vi "stop.vi"(8 "error in (no error)":errorcluster, 11 "SignalReaderCN091129DAQmx in":refnum<class "SignalReaderCN091129DAQmx.lvclass">) -> (0 "error out":errorcluster, 3 "SignalReaderCN091129DAQmx out":refnum<class "SignalReaderCN091129DAQmx.lvclass">)   [LabVIEW 2010, in "SignalReaderCN091129DAQmx.lvclass"]
uses:
  SignalReaderCN091129DAQmx.lvclass
  GenericSignalReader/GenericSignalReader/GenericSignalReader.lvclass
  SignalReaderCN091129DAQmx.lvclass/SignalReaderCN091129DAQmx.ctl
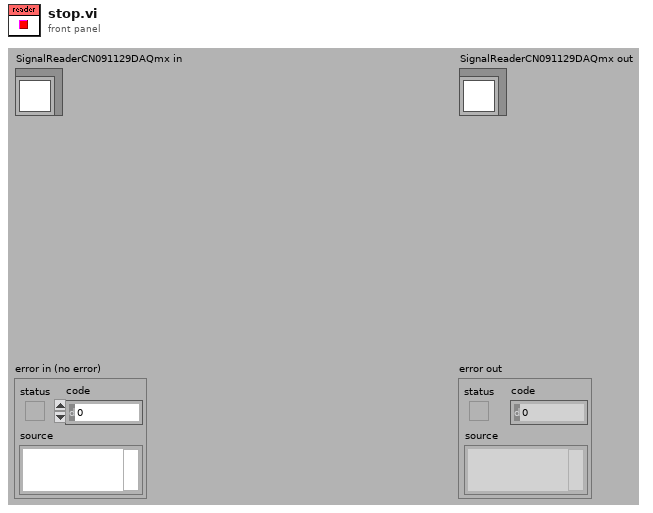
[diagram p1: front panel]
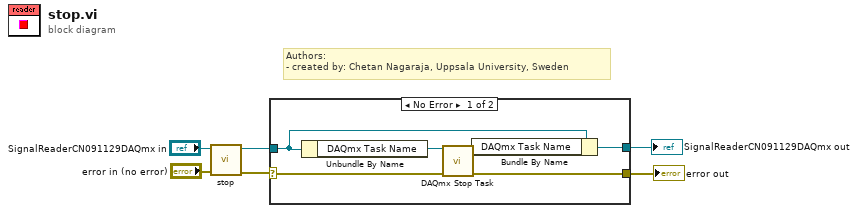
[diagram p0: block diagram]
diagram:
  # "Authors: \n- created by: Chetan Nagaraja, Uppsala University, Sweden"
  n1 = call-parent "stop.vi"("error in (no error)"="error in (no error)", "GenericSignalReader in"="SignalReaderCN091129DAQmx in") -> ("error out"=w4:errorcluster, "GenericSignalReader out"=w3:refnum<class "SignalReaderCN091129DAQmx.lvclass">)  [unwired: 8 in]
  n2 = case shown="No Error" w4 {
    selector: w4 -> [w12 w13]
    tunnel: w3 -> [w10 w14]
    tunnel: [w9 w14] -> w2
    tunnel: [w11 w13] -> w1
    frame No Error {
      n3 = Unbundle By Name(w10) -> ("DAQmx Task Name"=w8:refnum<k21>)
      n4 = call <vilib>:"DAQmx Stop Task.vi"("task/channels in"=w8, "error in"=w12) -> ("task out"=w7:refnum<k21>, "error out"=w11:errorcluster)  [unwired: 12 in]
      n5 = Bundle By Name(cluster=w10, "DAQmx Task Name"=w7) -> (w9:refnum<class "SignalReaderCN091129DAQmx.lvclass">)
    }
    frame Error {
    }
  }
  "error out" <- w1
  "SignalReaderCN091129DAQmx out" <- w2
